vi "Add Remove Test.vi"() -> (0 "error out":errorcluster, 2 "Success Delete":bool, 3 "Success ADD":bool)   [LabVIEW 2013, in "Scan Engine tests.lvlib"]
uses:
  Scan Engine tests.lvlib
  <vilib>/NI/Tag Bus/tag/Data Type.ctl
  configuration/Line.ctl
  <vilib>/NI/Tag Bus Module Framework/channel/TBM channel.lvclass
  editor node/permissions.ctl
  configuration/Scan Engine configuration.lvclass
  <vilib>/NI/Tag Bus/tag/tag descriptor.lvclass
  editor node/Scan Engine editor node.lvclass
panel:
  out "Deleted Line":string
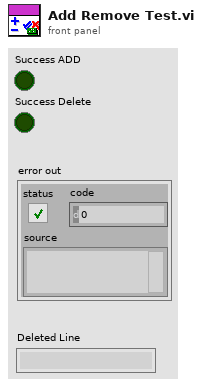
[diagram p1: front panel]
types:
  T1 = typedef "Scan Engine editor node.lvclass/permissions.ctl" = enum32{"Read from HW", "Write to HW"}
  T2 = typedef "Scan Engine configuration.lvclass/Line.ctl" = cluster{"channel":refnum<class "TBM channel.lvclass">, "Tag":string}
  T3 = typedef "tag bus.lvlib/tag descriptor.lvclass/Data Type.ctl" = enum16{"Double", "Single", "I64", "I32", "I16", "I8", "U64", "U32", "U16", "U8", "Boolean", "String", "Array of Double", "Array of Single", "Array of I64", "Array of I32", "Array of I16", "Array of I8", "Array of U64", "Array of U32", "Array of U16", "Array of U8", "Array of Boolean", "Array of String"}
  T4 = typedef "TBM channel.lvclass/channel classification.ctl" = enum16{"input data", "output data", "processing parameter", "processing result"}
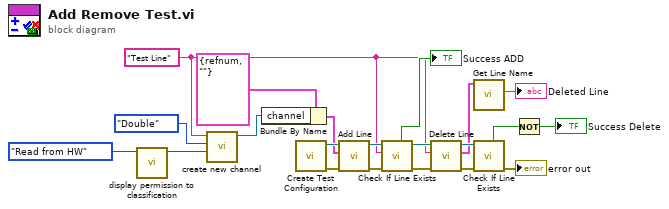
[diagram p0: block diagram]
diagram:
  w9 = "Test Line" ("channel name")
  n1 = call "display permission to classification.vi"("display permissions"=permissions."Read from HW") -> ("channel classification"=w19:T4)  [unwired: 10 in]
  n2 = call <vilib>:"create new channel.vi"("channel classification"=w19, "data type"=Data_Type."Double", "channel name"=w9) -> ("channel"=w20:refnum<class "TBM channel.lvclass">)  [unwired: 8 in]
  n3 = Bundle By Name(cluster=T2 {"channel"=refnum, "Tag"=""} ("Line"), "channel"=w20) -> (w17:T2)
  n4 = call "Create Test Configuration.vi"() -> ("error out"=w10:errorcluster, "module"=w21:refnum<class "Scan Engine configuration.lvclass">)  [unwired: 6 in, 4 out]
  n5 = call "Add Line.vi"("error in"=w10, "Line"=w17, "Scan Engine configuration in"=w21) -> ("error out"=w12:errorcluster, "Scan Engine configuration out"=w15:refnum<class "Scan Engine configuration.lvclass">)  [unwired: 7 in]
  n6 = call-dynamic "Check If Line Exists.vi"("error in"=w12, "name to locate"=w9, "Scan Engine configuration in"=w15) -> ("error out"=w11:errorcluster, "Scan Engine configuration out"=w14:refnum<class "Scan Engine configuration.lvclass">, "found?"=→"Success ADD":bool)  [unwired: 4 in, 2 out]
  n7 = call "Delete Line.vi"("error in"=w11, "Active Line Name"=w9, "Scan Engine configuration in"=w14) -> ("error out"=w8:errorcluster, "deleted line"=w2:T2, "Scan Engine configuration out"=w6:refnum<class "Scan Engine configuration.lvclass">)  [unwired: 6 in]
  n8 = call "Get Line Name.vi"("Line in"=w2) -> ("Name"=→"Deleted Line":string)  [unwired: 8 in, 2 out]
  n9 = call-dynamic "Check If Line Exists.vi"("error in"=w8, "Scan Engine configuration in"=w6) -> ("error out"=→"error out":errorcluster, "found?"=w5:bool)  [unwired: 5 in, 3 out]
  n10 = Not(x=w5) -> (.not. x?=→"Success Delete":bool)
